vi "PH_AWG-510.PC Set Expert Mode.vi"(0 "VI in":refnum<vi>, 2 "Expert Mode":bool, 5 "error in (no error)":errorcluster) -> (14 "VI out":refnum<vi>, 19 "error out":errorcluster)   [LabVIEW 2014, in "PH_AWG-510.lvlib"]
uses:
  PH_AWG-510.lvlib
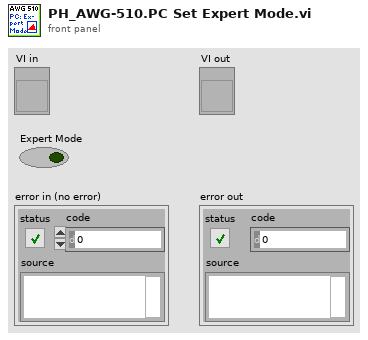
[diagram p1: front panel]
types:
  T1 = typedef "PH_AWG-510.lvlib/PH_AWG-510.i attribute.ctl" = cluster{"GUI Refs":cluster{"Delete":refnum<vi>, "Trigger Settings":refnum<vi>, "Start Device":refnum<vi>, "Instrument Information":refnum<vi>, "Lock Frontpanel":refnum<vi>, "Waveform Pattern File":refnum<vi>, "Initialize":refnum<vi>, "Output Settings":refnum<vi>}, "Instrument Information":T2, "Initialized?":bool, "Current Settings":cluster{"Trigger":T3, "Output Settings":T4}, "Wanted Settings":cluster{"Trigger":T3, "Output Settings":T4}, "Device frontpanel locked?":bool, "Default File Path":path}
  T2 = typedef "PH_AWG-510.lvlib/PH_AWG-510.Instrument Information Dataset.ctl" = cluster{"VISA resource name":refnum<visa-resource-name>, "Instrument Firmware Revision":string, "Manufacturer":string, "Model":string, "Serial Number":string, "Error Message":string, "Device Status":enum16{"stopped", "wating for trigger", "running", "Failure"}}
  T3 = typedef "PH_AWG-510.lvlib/PH_AWG-510.Trigger Settings.ctl" = cluster{"Mode":enum16{"Continuous", "Triggered", "Gated", "Enhanced"}, "Level (V)":dbl, "External Source":bool}
  T4 = typedef "PH_AWG-510.lvlib/PH_AWG-510.Output Settings.ctl" = cluster{"Activate Channel":bool, "VPP (V)":dbl, "Clock (Hz)":dbl, "File Name (Device)":string, "#1":u16, "#2":u16, "#3":u16, "#4":u16, "#5":u16, "#6":u16, "#7":u16, "#8":u16, "#9":u16, "#10":u16, "#11":u16, "#12":u16, "#13":u16, "#14":u16, "#15":u16, "#16":u16, "#17":u16, "#18":u16, "#19":u16, "#20":u16, "Offset (V)":dbl}
  T5 = enum8{"Enabled", "Disabled", "Disabled and Grayed Out"}
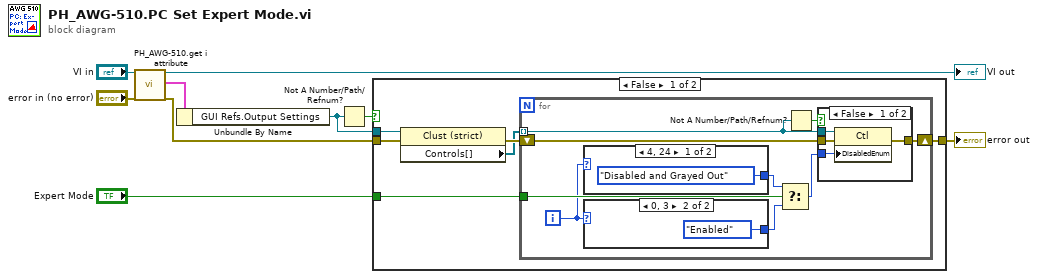
[diagram p0: block diagram]
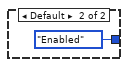
[diagram p2: hidden frame]
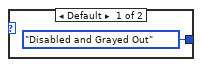
[diagram p3: hidden frame]
diagram:
  n1 = call "PH_AWG-510.get i attribute.vi"("i ref in"="VI in", "error in (no error)"="error in (no error)") -> ("i ref out"=→"VI out":refnum<vi>, "i attribute"=w5:T1, "error out"=w9:errorcluster)  [unwired: 15 in]
  n2 = Unbundle By Name(w5) -> ("GUI Refs.Output Settings"=w1:refnum<vi>)
  n3 = Not A Number/Path/Refnum?(number/path/refnum=w1) -> (NaN/Path/Refnum?=w2:bool)
  n4 = case shown="False" w2 {
    tunnel: w9 -> [w15 w34]
    tunnel: w1 -> [w14 _]
    tunnel: [w12 w34] -> w4
    tunnel: "Expert Mode" -> [w10 _]
    frame False {
      n5 = property class="Clust (strict)"(reference=w14, error in=w15) -> (error out=w13:errorcluster, "Controls[]"=w11:refnum<vi>[])  [unwired: 1 out]
      n6 = for {
        shift-right: [w23] -> w12
        shift-left: w13 -> [w24]
        tunnel: w11 -> [w21] mode=indexing
        tunnel: w10 -> [w20]
        i -> [w16]
        n7 = case shown="4, 24" w16 {
          tunnel: [T5."Disabled and Grayed Out" ("Disabled") T5."Enabled" ("Disabled")] -> w17
          frame 4, 24 {
          }
          frame Default {
          }
        }
        n8 = case shown="0, 3" w16 {
          tunnel: [T5."Disabled and Grayed Out" ("Disabled") T5."Enabled" ("Disabled")] -> w19
          frame Default {
          }
          frame 0, 3 {
          }
        }
        n9 = Select(t=w17, s=w20, f=w19) -> (s? t:f=w18:T5)
        n10 = Not A Number/Path/Refnum?(number/path/refnum=w21) -> (NaN/Path/Refnum?=w22:bool)
        n11 = case shown="False" w22 {
          tunnel: w24 -> [w32 w33]
          tunnel: [w31 w33] -> w23
          tunnel: w21 -> [w30 _]
          tunnel: w18 -> [w29 _]
          frame False {
            n12 = property class="Ctl"(reference=w30, error in=w32, "DisabledEnum"=w29) -> (error out=w31:errorcluster)  [unwired: 1 out]
          }
          frame True {
          }
        }
      }
    }
    frame True {
    }
  }
  "error out" <- w4
